vi "ReadData.vi"(8 "error in (no error)":errorcluster, 11 "Communication in":refnum<class "Communication.lvclass">) -> (0 "error out":errorcluster, 2 "read buffer":string, 3 "Communication out":refnum<class "Communication.lvclass">)   [LabVIEW 2019, in "Communication.lvclass"]
uses:
  Communication.lvclass
  Communication.lvclass/Communication.ctl
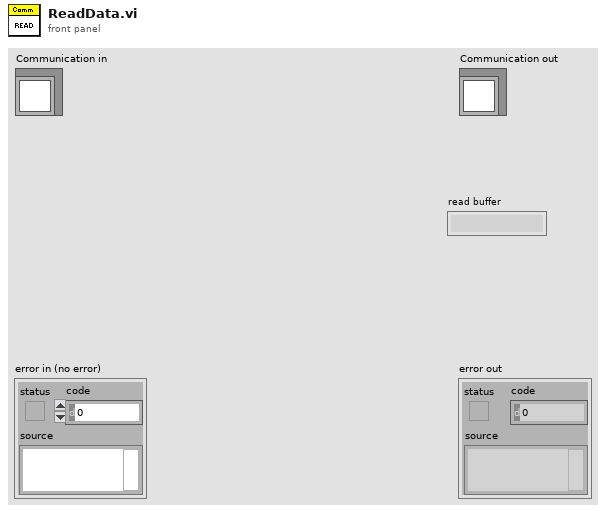
[diagram p1: front panel]
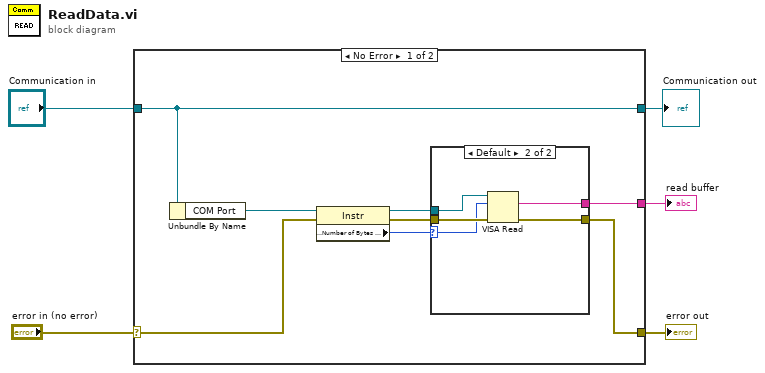
[diagram p0: block diagram]
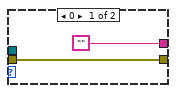
[diagram p2: hidden frame]
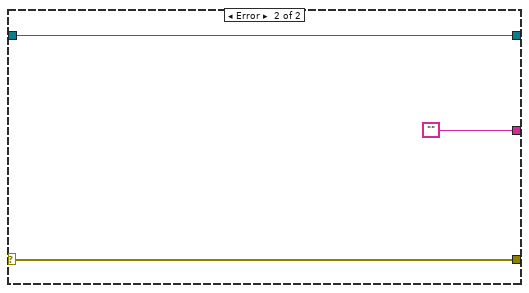
[diagram p3: hidden frame]
diagram:
  n1 = case shown="No Error" "error in (no error)" {
    selector: "error in (no error)" -> [w12 w23]
    tunnel: [w8 w23] -> w4
    tunnel: [w6 w22] -> w2
    tunnel: "Communication in" -> [w6 w22]
    tunnel: [w7 ""] -> w1
    frame No Error {
      n2 = Unbundle By Name(w6) -> ("COM Port"=w13:refnum<visa-resource-name>)
      n3 = property class="Instr"(reference=w13, error in=w12) -> (reference out=w11:refnum<visa-resource-name>, error out=w9:errorcluster, "Serial Settings:Number of Bytes at Serial Port"=w10:u32)
      n4 = case shown="Default" w10 {
        selector: w10 -> [_ w16]
        tunnel: w11 -> [_ w20]
        tunnel: w9 -> [w14 w19]
        tunnel: [w14 w18] -> w8
        tunnel: ["" w17] -> w7
        frame 0 {
        }
        frame Default {
          n5 = VISA Read(VISA resource name=w20, byte count=w16, error in (no error)=w19) -> (read buffer=w17:string, error out=w18:errorcluster)  [unwired: 2 out]
        }
      }
    }
    frame Error {
    }
  }
  "error out" <- w4
  "Communication out" <- w2
  "read buffer" <- w1
